vi "recallMovesOnRobot.vi"(0 "Plan":string, 3 "error in (no error)":errorcluster) -> (7 "Array":T1[](array[typedef]), 10 "error IO":errorcluster)   [LabVIEW 2018]
uses:
  Drive Auton.ctl
panel:
  out "path 2":path
  out "path":path
  in  "Path":string="/home/lvuser/config/"
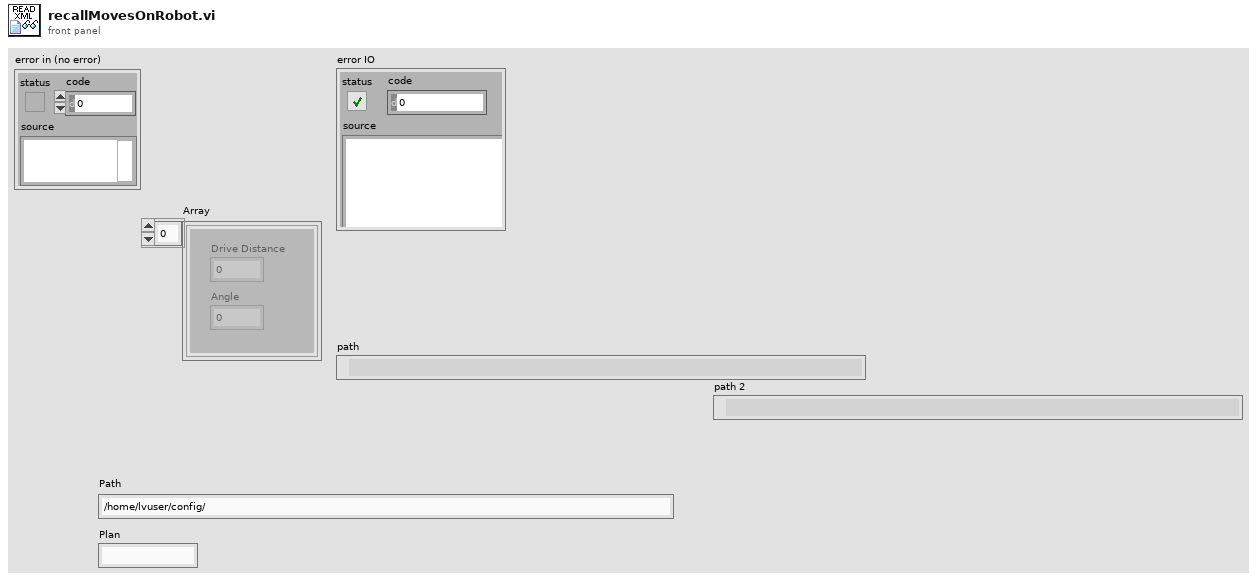
[diagram p1: front panel]
types:
  T1 = typedef "Drive Auton.ctl" = cluster{"Drive Distance":dbl, "Angle":dbl}
  T2 = enum16{"open", "replace", "create", "open or create", "replace or create", "replace or create with confirmation"}
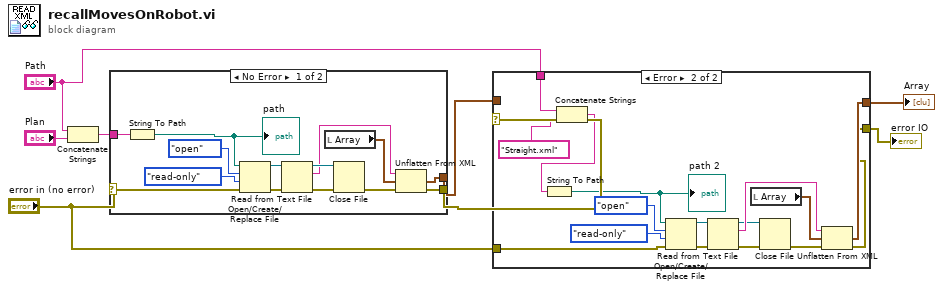
[diagram p0: block diagram]
diagram:
  n1 = Concatenate Strings("Path", "Plan") -> (w7:string)
  n2 = case shown="No Error" "error in (no error)" {
    selector: "error in (no error)" -> [w20 w23]
    tunnel: w7 -> [w22 _]
    tunnel: [w10 w23] -> w6
    tunnel: [w9 _] -> w5
    frame No Error {
      n3 = String To Path(string=w22) -> (path=w21:path)
      "path" <- w21
      n4 = Open/Create/Replace File(file path (use dialog)=w21, error in=w20, operation (0:open)=T2."open", access (0:read/write)=enum16{"read/write", "read-only", "write-only"}."read-only") -> (refnum out=w17:refnum<file>, error out=w15:errorcluster)  [unwired: 2 in, 1 out]
      n5 = Read from Text File(file (use dialog)=w17, error in=w15) -> (refnum out=w16:refnum<file>, text=w13:string, error out=w14:errorcluster)  [unwired: 2 in, 1 out]
      n6 = local read "Array"() -> (w12:T1[])
      n7 = Close File(refnum=w16, error in=w14) -> (error out=w11:errorcluster)  [unwired: 1 out]
      n8 = Unflatten From XML(xml string=w13, type=w12, error in (no error)=w11) -> (value=w9:T1[], error out=w10:errorcluster)
    }
    frame Error {
    }
  }
  n9 = case shown="Error" w6 {
    selector: w6 -> [w24 _]
    tunnel: w5 -> [w25 _]
    tunnel: [w25 w28] -> w4
    tunnel: [w24 w27] -> w3
    tunnel: "Path" -> [_ w31]
    tunnel: "error in (no error)" -> [_ w26]
    frame No Error {
    }
    frame Error {
      n10 = Concatenate Strings(w31, "Straight.xml") -> (w29:string)
      n11 = String To Path(string=w29) -> (path=w32:path)
      "path 2" <- w32
      n12 = Open/Create/Replace File(file path (use dialog)=w32, error in=w26, operation (0:open)=T2."open", access (0:read/write)=enum16{"read/write", "read-only", "write-only"}."read-only") -> (refnum out=w35:refnum<file>, error out=w37:errorcluster)  [unwired: 2 in, 1 out]
      n13 = Read from Text File(file (use dialog)=w35, error in=w37) -> (refnum out=w36:refnum<file>, text=w39:string, error out=w38:errorcluster)  [unwired: 2 in, 1 out]
      n14 = local read "Array"() -> (w40:T1[])
      n15 = Close File(refnum=w36, error in=w38) -> (error out=w41:errorcluster)  [unwired: 1 out]
      n16 = Unflatten From XML(xml string=w39, type=w40, error in (no error)=w41) -> (value=w28:T1[], error out=w27:errorcluster)
    }
  }
  "Array" <- w4
  "error IO" <- w3
